vi "Clear Prompt Active.vi"(8 "error in (no error)":errorcluster, 11 "GUI Element in":refnum<class "GUI Element.lvclass">) -> (0 "error out":errorcluster, 3 "GUI Element out":refnum<class "GUI Element.lvclass">)   [LabVIEW 2020, in "VolatusGUI.lvlib" / "GUI Element.lvclass"]
uses:
  GUI Element.lvclass
  GUI Element.lvclass/GUI Element.ctl
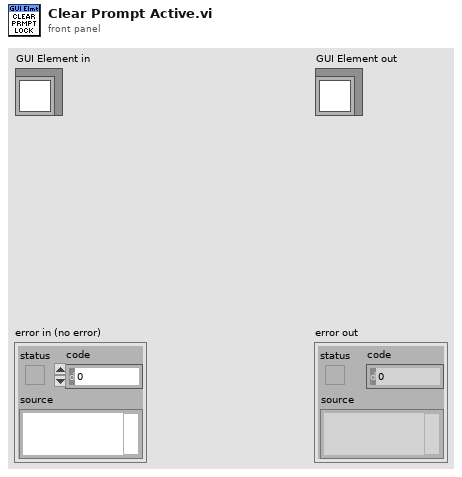
[diagram p1: front panel]
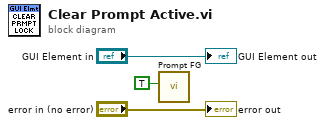
[diagram p0: block diagram]
diagram:
  n1 = call "Prompt FG.vi"("Clear"=TRUE) -> ()  [unwired: 10 in, 1 out]
  "error out" <- "error in (no error)"
  "GUI Element out" <- "GUI Element in"
